vi "Acquire.vi"(4 "# of pretrigger":u32, 5 "Circular Buffer Mem":refnum<k21>, 6 "Simulate":bool, 7 "Command FIFO":refnum<k21>, 8 "Records to Acquire":u32=300, 9 "Trigger":i16=100, 10 "FPGA I/O In":refnum<k21>="IO Module\\AI A0", 11 "Ch Armed Reg":refnum<k21>="Register 1") -> ()   [LabVIEW 2012]
uses:
  <vilib>/rvi/DataTransferAndStorage/Container/Common/niFpgaContainerExecOnDevCompGetState.vi
  <vilib>/rvi/Memory/Memory_Emulation/nirvimemoryEmulationManagerCache_GetValue.vi
  <vilib>/rvi/Memory/Memory_Emulation/niFpgaMemoryEmulationValidateCache.vi
  <vilib>/rvi/DataTransferAndStorage/Container/Common/niFpgaContainerGetUniqueNameForEmu.vi
  <vilib>/rvi/Memory/Memory_Emulation/nirvimemoryEmulationManagerCache_InsertValue.vi
  <vilib>/rvi/eio/common/nirviEmuTemplateMethod_errors.vi
  <vilib>/rvi/Emulation/niFpgaSctlEmulationGetInTimedLoop.vi
  <vilib>/rvi/FIFO/Fifo_Resource/nirvififoEmulationSetSize.vi
  <vilib>/rvi/errors/niFpgaSetErrorForExecOnDevCompSimple.vi
  <vilib>/rvi/eio/common/nirviEmuReportErrorAndStop.vi
  <vilib>/rvi/Emulation/niFpgaSctlEmulationFifoFullMgr.vi
  <vilib>/rvi/Emulation/niFpgaSctlEmulationResourceMgr.vi
  <vilib>/rvi/interface/RandomDataEmulation/nirviRandomDataFPGAFIFO.vi
  <vilib>/rvi/interface/RandomDataEmulation/niFpgaRandomDataHandleErrors.vi
  <vilib>/rvi/DataTransferAndStorage/Container/XNode/niFpgaContainer.xnode
  <vilib>/rvi/DataTransferAndStorage/Register/Emulation/niFpgaRegisterEmulationRefIn.vi
  <vilib>/eio/EIONode/EIONode.xnode
  <vilib>/rvi/FIFO/Fifo_Resource/niFpgaFifoEmulationRefIn.vi
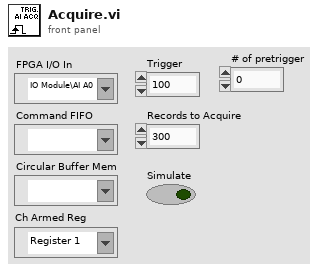
[diagram p1: front panel]
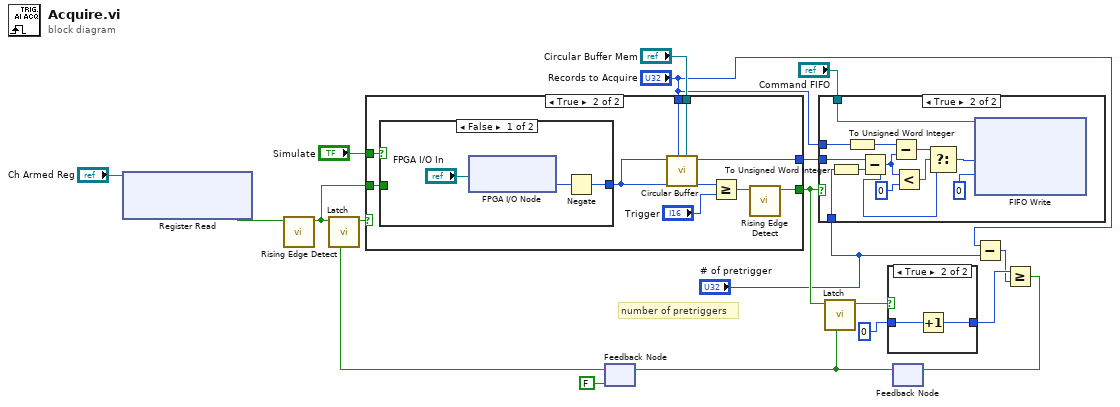
[diagram p0: block diagram]
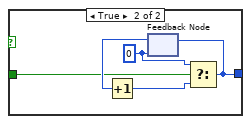
[diagram p4: hidden frame]
diagram:
  # "number of pretriggers"
  n1 = xnode ("Register Read")("Register In"="Ch Armed Reg") -> ("Data"=w13:bool)  [unwired: 1 out]
  n2 = call "Rising Edge Detect.vi"("Input"=w13) -> ("Rising Edge"=w11:bool)  [unwired: 10 in]
  n3 = feedback #1(FALSE) -> (w14:bool)
  n4 = call "Latch.vi"("Reset"=w14, "Input"=w11) -> ("Output"=w15:bool)  [unwired: 9 in]
  n5 = case shown="True" w15 {
    tunnel: "Circular Buffer Mem" -> [_ w28]
    tunnel: [_ w22] -> w9
    tunnel: "Records to Acquire" -> [_ w25]
    tunnel: [_ w24] -> w17
    tunnel: w11 -> [_ w21]
    tunnel: "Simulate" -> [_ w20]
    frame False {
    }
    frame True {
      n6 = case shown="False" w20 {
        tunnel: [w29 w33] -> w27
        tunnel: w21 -> [_ w32]
        frame False {
          n7 = xnode "FPGA I/O Node"("FPGA I/O In"="FPGA I/O In") -> ("I/O Item"=w31:i16)  [unwired: 1 out]
          n8 = Negate(x=w31) -> (-x=w29:i16)
        }
        frame True {
          w34 = i16 0 ("x")
          n9 = feedback #2(w34) -> (w36:i16)
          n10 = Increment(x=w36) -> (x+1=w35:i16)
          n11 = Select(t=w34, s=w32, f=w35) -> (s? t:f=w33:i16)
          n12 = feedback-in #2(w33) -> ()
        }
      }
      n13 = call "Circular Buffer.vi"("Refnum in"=w28, "Records to Acquire"=w25, "Data"=w27) -> ("Address"=w24:u16)  [unwired: 8 in]
      n14 = Greater Or Equal?(x=w27, y="Trigger") -> (x >= y?=w23:bool)
      n15 = call "Rising Edge Detect.vi"("Input"=w23) -> ("Rising Edge"=w22:bool)  [unwired: 10 in]
    }
  }
  n16 = case shown="True" w9 {
    tunnel: "Command FIFO" -> [_ w48]
    tunnel: w17 -> [_ w46]
    tunnel: "# of pretrigger" -> [_ w45]
    tunnel: "Records to Acquire" -> [_ w39]
    frame False {
    }
    frame True {
      n17 = To Unsigned Word Integer(number=w45) -> (unsigned 16bit integer=w44:u16)
      n18 = To Unsigned Word Integer(number=w39) -> (unsigned 16bit integer=w38:u16)
      n19 = Subtract(x=w46, y=w44) -> (x-y=w40:u16)
      n20 = Subtract(x=w38, y=w40) -> (x-y=w41:u16)
      n21 = Less?(x=w40, y=u16 0) -> (x < y?=w43:bool)
      n22 = Select(t=w41, s=w43, f=w40) -> (s? t:f=w37:u16)
      n23 = xnode ("FIFO Write")("Element"=w37, "Timeout"=0, "FIFO In"=w48) -> ()  [unwired: 2 out]
    }
  }
  n24 = feedback #3() -> (w3:bool)  [unwired: 1 in]
  n25 = feedback-in #1(w3) -> ()
  n26 = call "Latch.vi"("Reset"=w3, "Input"=w9) -> ("Output"=w8:bool)  [unwired: 9 in]
  n27 = case shown="True" w8 {
    tunnel: u32 0 -> [w49 w51]
    tunnel: [w49 w50] -> w6
    frame False {
    }
    frame True {
      n28 = Increment(x=w51) -> (x+1=w50:u32)
    }
  }
  n29 = Subtract(x="Records to Acquire", y="# of pretrigger") -> (x-y=w5:u32)
  n30 = Greater Or Equal?(x=w6, y=w5) -> (x >= y?=w4:bool)
  n31 = feedback-in #3(w4) -> ()
